vi "nipkg-updateControlFileDescription.vi"(8 "error in (no error)":errorcluster, 10 "New Package Description":string, 11 "Package data":T1) -> (0 "error out":errorcluster, 3 "Package data out":T1)   [LabVIEW 2014, in "nipkg-build-system.lvlib"]
uses:
  nipkg-build-system.lvlib
  types/Package data.ctl
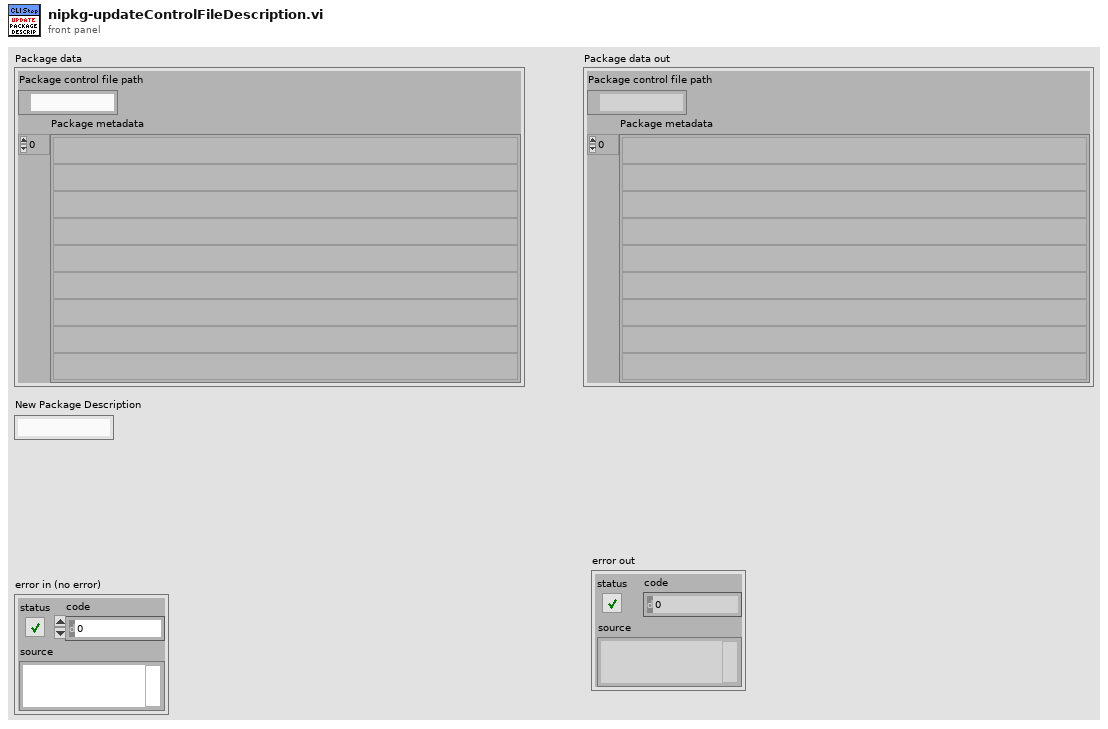
[diagram p1: front panel]
types:
  T1 = typedef "nipkg-build-system.lvlib/Package data.ctl" = cluster{"Package control file path":path, "Package metadata":string[]}
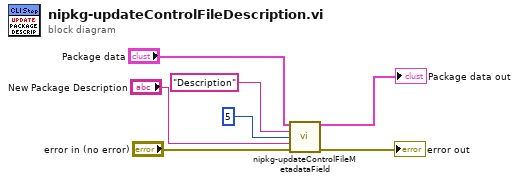
[diagram p0: block diagram]
diagram:
  n1 = call "nipkg-updateControlFileMetadataField.vi"("Package data"="Package data", "Metadata field name"="Description", "Metadata field index"=u8 5, "Metadata field value"="New Package Description", "error in (no error)"="error in (no error)") -> ("Package data out"=→"Package data out":T1, "error out"=→"error out":errorcluster)  [unwired: 9 in]
